vi "AutoPressA.vi"(1 "Time Since Latch":u32, 2 "Instruction String":string) -> (0 "Advance Trigger":bool)   [LabVIEW 2019]
uses:
  dsinstructions.vi
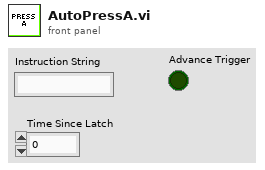
[diagram p1: front panel]
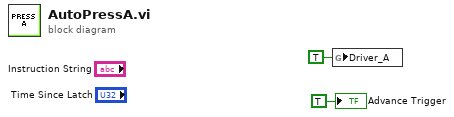
[diagram p0: block diagram]
diagram:
  n1 = global write "dsinstructions.vi" "Driver_A"(TRUE ("Driver_A")) -> ()
  "Advance Trigger" <- TRUE ("Advance Trigger")
